vi "IRTransmitRaw.vi"(0 "Device In":u64, 5 "carrierFrequency":u32, 7 "gap":u32, 9 "Data":u32[](array[numeric]), 11 "error in (no error)":errorcluster, 12 "dutyCycle":dbl) -> (4 "Device Out":u64, 15 "error out":errorcluster)   [LabVIEW 2012, in "Phidget IR.lvlib"]
doc: "${TransmitRaw:Header}"
uses:
  <instrlib>/Phidgets/Phidget IR/Phidget IR.lvlib
  <instrlib>/Phidgets/Phidget Common/Phidget Common.lvlib
  phidget22.dll
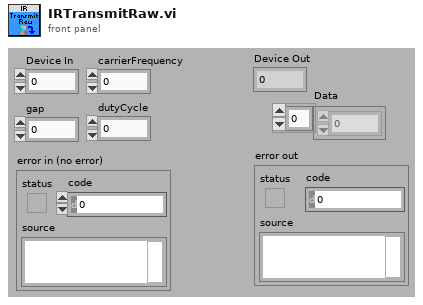
[diagram p1: front panel]
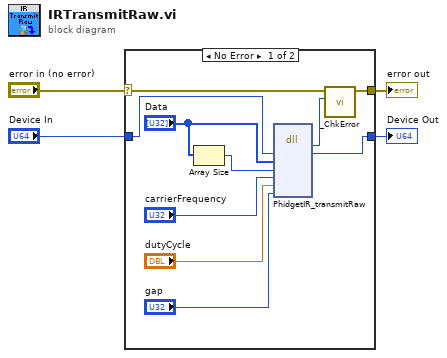
[diagram p0: block diagram]
diagram:
  n1 = case shown="No Error" "error in (no error)" {
    selector: "error in (no error)" -> [w13 w16]
    tunnel: [w12 w16] -> w3
    tunnel: "Device In" -> [w11 w15]
    tunnel: [w10 w15] -> w1
    frame No Error {
      n2 = Array Size(array="Data") -> (size(s)=w5:i32)
      n3 = dll-call lib="phidget22.*" fn="PhidgetIR_transmitRaw"("phid"=w11, "data"="Data", "length"=w5, "carrierFrequency"="carrierFrequency", "dutyCycle"="dutyCycle", "gap"="gap") -> ("return type"=w14:i32, "phid"=w10:u64)  [unwired: 8 in, 2 out]
      n4 = call <instrlib>:"_ChkError.vi"("Return Code"=w14, "error in (no error)"=w13) -> ("error out"=w12:errorcluster)  [unwired: 9 in]
    }
    frame Error {
    }
  }
  "error out" <- w3
  "Device Out" <- w1
